vi "get_single_acq.vi"(8 "error in (no error)":errorcluster, 11 "glaz in":refnum<class "glaz.lvclass">) -> (0 "error out":errorcluster, 1 "trigger":bool[][](array[boolean]), 2 "raw data":i32[][][](array[numeric]), 3 "glaz out":refnum<class "glaz.lvclass">)   [LabVIEW 2019, in "glaz.lvlib" / "glaz.lvclass"]
uses:
  glaz.lvclass
  D:/github/TransientAbsorptionDAQ.lv/_camera/_camera.lvlibp/_cameraClass/_camera.lvclass
  _camera/_camera.lvlibp/_cameraClass/Read background.vi
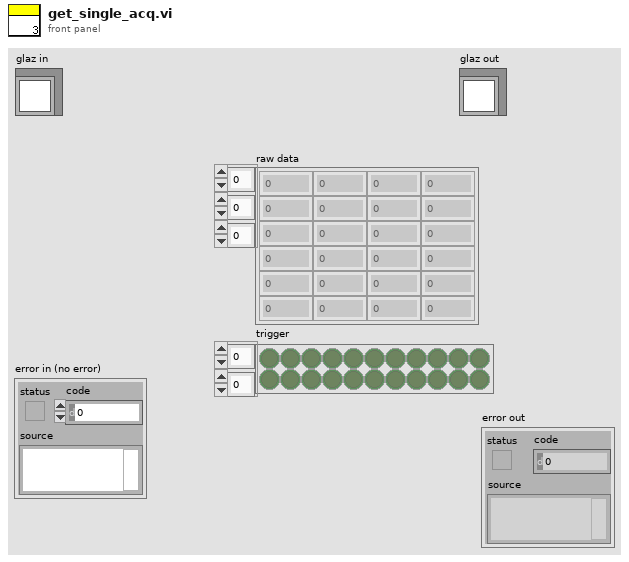
[diagram p1: front panel]
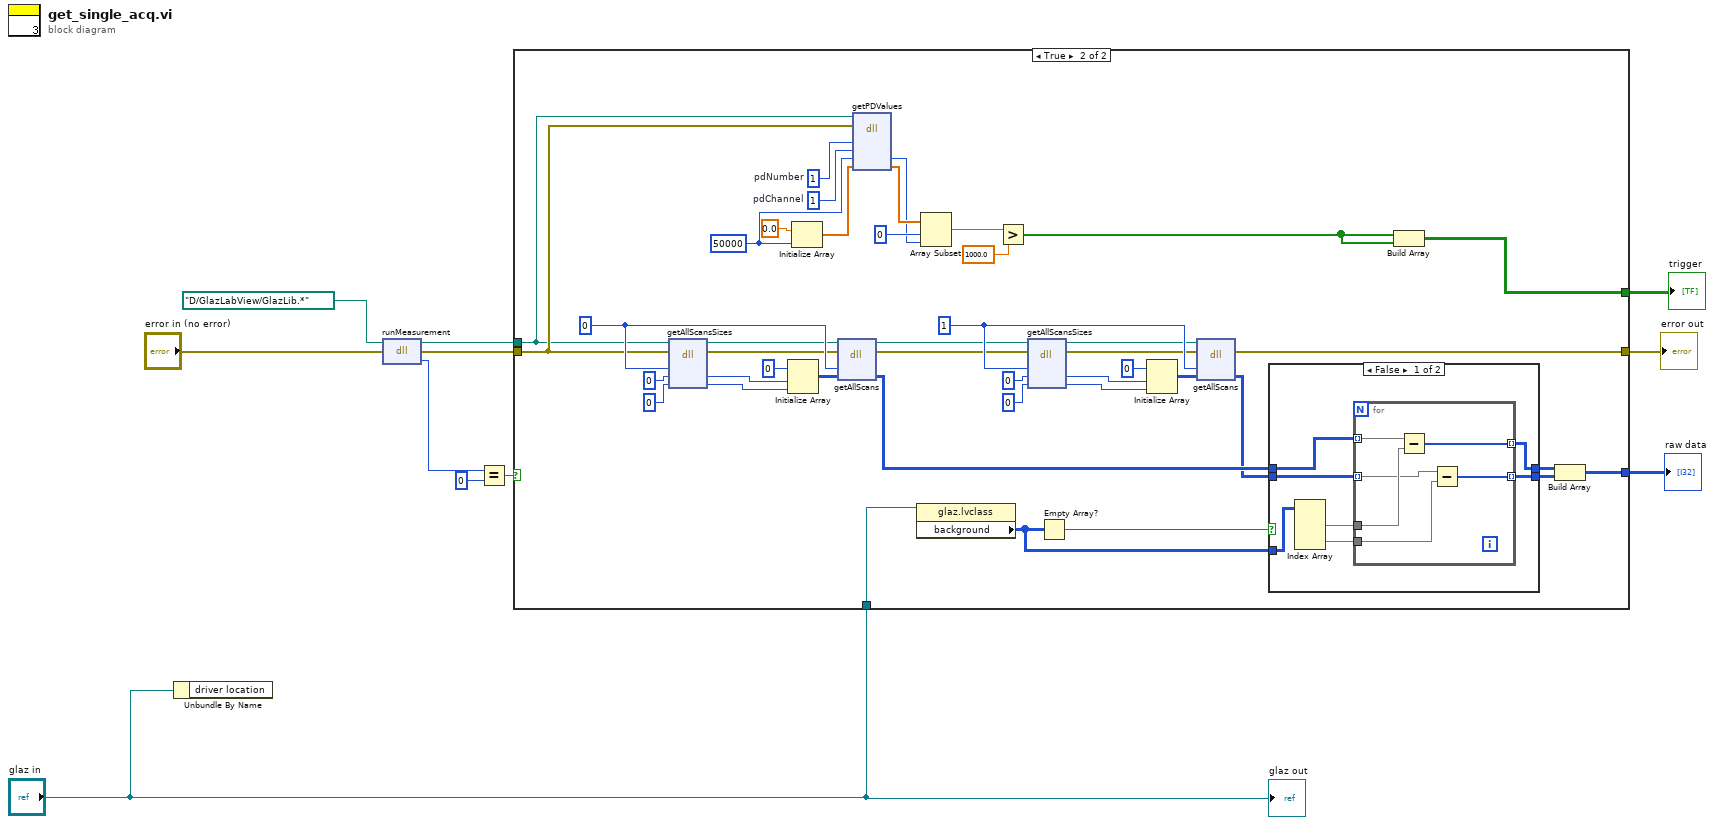
[diagram p0: block diagram]
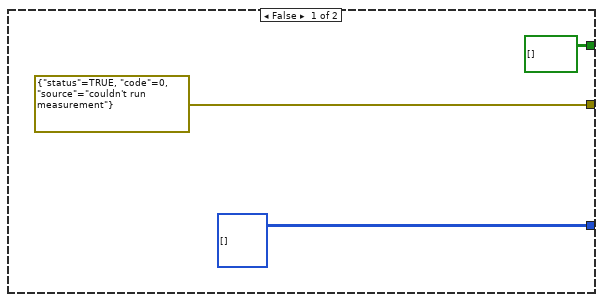
[diagram p2: hidden frame]
diagram:
  n1 = Unbundle By Name("glaz in") -> ()  [unwired: 1 out]
  n2 = dll-call lib="C:/Program Files/National Instruments/LabVIEW 2019/user.lib/GlazLabView/GlazLib.*" fn="runMeasurement"(path in=path "D:/GlazLabView/GlazLib.*", error in="error in (no error)") -> (path out=w6:path, error out=w8:errorcluster, "return type"=w4:i32)  [unwired: 1 in]
  n3 = Equal?(x=w4, y=0) -> (x = y?=w5:bool)
  n4 = case shown="True" w5 {
    tunnel: [u16[][][] [] w40] -> w11
    tunnel: [errorcluster {"status"=TRUE, "code"=0, "source"="couldn't run measurement"} ("error out") w28] -> w10
    tunnel: w8 -> [_ w19]
    tunnel: w6 -> [_ w18]
    tunnel: "glaz in" -> [_ w36]
    tunnel: [bool[][] [] w29] -> w2
    frame False {
    }
    frame True {
      w26 = 1  # pdChannel
      w27 = 1  # pdNumber
      w25 = 50000 ("count")
      w49 = 1 ("calculationIndex")
      w57 = 0 ("calculationIndex")
      n5 = dll-call lib="C:/Program Files/National Instruments/LabVIEW 2019/user.lib/GlazLabView/GlazLib.*" fn="getAllScansSizes"(path in=w18, error in=w19, "calculationIndex"=w57, "rowCount"=0, "coloumnCount"=0) -> (path out=w39:path, error out=w50:errorcluster, "rowCount"=w54:i32, "coloumnCount"=w55:i32)  [unwired: 3 in]
      n6 = Initialize Array(u16 0 ("element"), w54, w55) -> (w56:u16[][])
      n7 = Initialize Array(0.0 ("element"), w25) -> (w24:dbl[])
      n8 = dll-call lib="C:/Program Files/National Instruments/LabVIEW 2019/user.lib/GlazLabView/GlazLib.*" fn="getAllScans"(path in=w39, error in=w50, "calculationIndex"=w57, "values"=w56) -> (path out=w38:path, error out=w41:errorcluster, "values"=w34:u16[][])  [unwired: 3 in]
      n9 = dll-call lib="C:/Program Files/National Instruments/LabVIEW 2019/user.lib/GlazLabView/GlazLib.*" fn="getPDValues"(path in=w18, error in=w19, "pdNumber"=w27, "pdChannel"=w26, "count"=w25, "values"=w24) -> ("count"=w20:i32, "values"=w22:dbl[])  [unwired: 4 in, 2 out]
      n10 = property class="glaz.lvclass"(reference=w36) -> ("background"=w33:i32[][])  [unwired: 1 in, 2 out]
      n11 = Array Subset(array=w22, index=0, length=w20) -> (w17:dbl[])
      n12 = Greater?(x=w17, y=1000.0) -> (0:w15:bool[])
      n13 = dll-call lib="C:/Program Files/National Instruments/LabVIEW 2019/user.lib/GlazLabView/GlazLib.*" fn="getAllScansSizes"(path in=w38, error in=w41, "calculationIndex"=w49, "rowCount"=0, "coloumnCount"=0) -> (path out=w37:path, error out=w42:errorcluster, "rowCount"=w46:i32, "coloumnCount"=w47:i32)  [unwired: 3 in]
      n14 = Empty Array?(array=w33) -> (empty?=w35:bool)
      n15 = Initialize Array(u16 0 ("element"), w46, w47) -> (w48:u16[][])
      n16 = dll-call lib="C:/Program Files/National Instruments/LabVIEW 2019/user.lib/GlazLabView/GlazLib.*" fn="getAllScans"(path in=w37, error in=w42, "calculationIndex"=w49, "values"=w48) -> (error out=w28:errorcluster, "values"=w31:u16[][])  [unwired: 3 in, 1 out]
      n17 = case shown="False" w35 {
        tunnel: w34 -> [w63 w72]
        tunnel: w33 -> [w64 _]
        tunnel: [w58 w72] -> w32
        tunnel: w31 -> [w61 w71]
        tunnel: [w59 w71] -> w30
        frame False {
          n18 = Index Array(array=w64) -> (element #1=w62:i32[], element #2=w60:i32[])  [unwired: 4 in]
          n19 = for {
            tunnel: w63 -> [w70] mode=indexing
            tunnel: w62 -> [w69]
            tunnel: w61 -> [w68] mode=indexing
            tunnel: w60 -> [w67]
            tunnel: [w66] -> w59 mode=indexing
            tunnel: [w65] -> w58 mode=indexing
            n20 = Subtract(x=w70, y=w69) -> (x-y=w65:i32[])
            n21 = Subtract(x=w68, y=w67) -> (x-y=w66:i32[])
          }
        }
        frame True {
        }
      }
      n22 = Build Array(w15, w15) -> (w29:bool[][])
      n23 = Build Array(w32, w30) -> (w40:i32[][][])
    }
  }
  "error out" <- w10
  "raw data" <- w11
  "trigger" <- w2
  "glaz out" <- "glaz in"
